vi "LJM logger write program config.vi"(0 "Working Directory":path, 7 "filename":string="ljstreamud.cfg", 9 "Program Configs":T1={"Data File Prefix"="", "Scan Rate (Hz)"=0.0, "Graph History"=0, "# Channels"=0, "Disable Scaling"=FALSE, "Max File Size (Bytes)"=0, "Channel Setup"={"Name"=["AIN0", "AIN1", "AIN2", "AIN3", "AIN4", "AIN5", "AIN6", "AIN7", "AIN8", "AIN9", "AIN10", "AIN11", "AIN12", "AIN13", "AIN14", "AIN15"], "", "Scaling Equation"=["y=a", "y=b", "y=c", "y=d", "y=e", "y=f", "y=g", "y=h", "y=i", "y=j", "y=k", "y=l", "y=m", "y=n", "y=o", "y=p"], "", "Graph?"=[TRUE, TRUE, TRUE, TRUE, FALSE, FALSE, FALSE, FALSE, FALSE, FALSE, FALSE, FALSE, FALSE, FALSE, FALSE, FALSE]}, "Interval (ms)"=0, "Write To File"=FALSE, "Log Every n Scans"=0}, 13 "Resolution":u8, 14 "SettlingFactor":u8) -> (15 "error out":errorcluster)   [LabVIEW 2026]
uses:
  Common Logger Controls/Program Config Cluster.ctl
  Common Logger Controls/Channel Setup.ctl
  <vilib>/Utility/config.llb/Write Key (String).vi
  <vilib>/Utility/config.llb/Write Key (I32).vi
  <vilib>/Utility/config.llb/Write Key (U32).vi
  <vilib>/Utility/config.llb/Write Key (Double).vi
  <vilib>/Utility/config.llb/Write Key (Boolean).vi
  <vilib>/Utility/config.llb/NI_LVConfig.lvlib
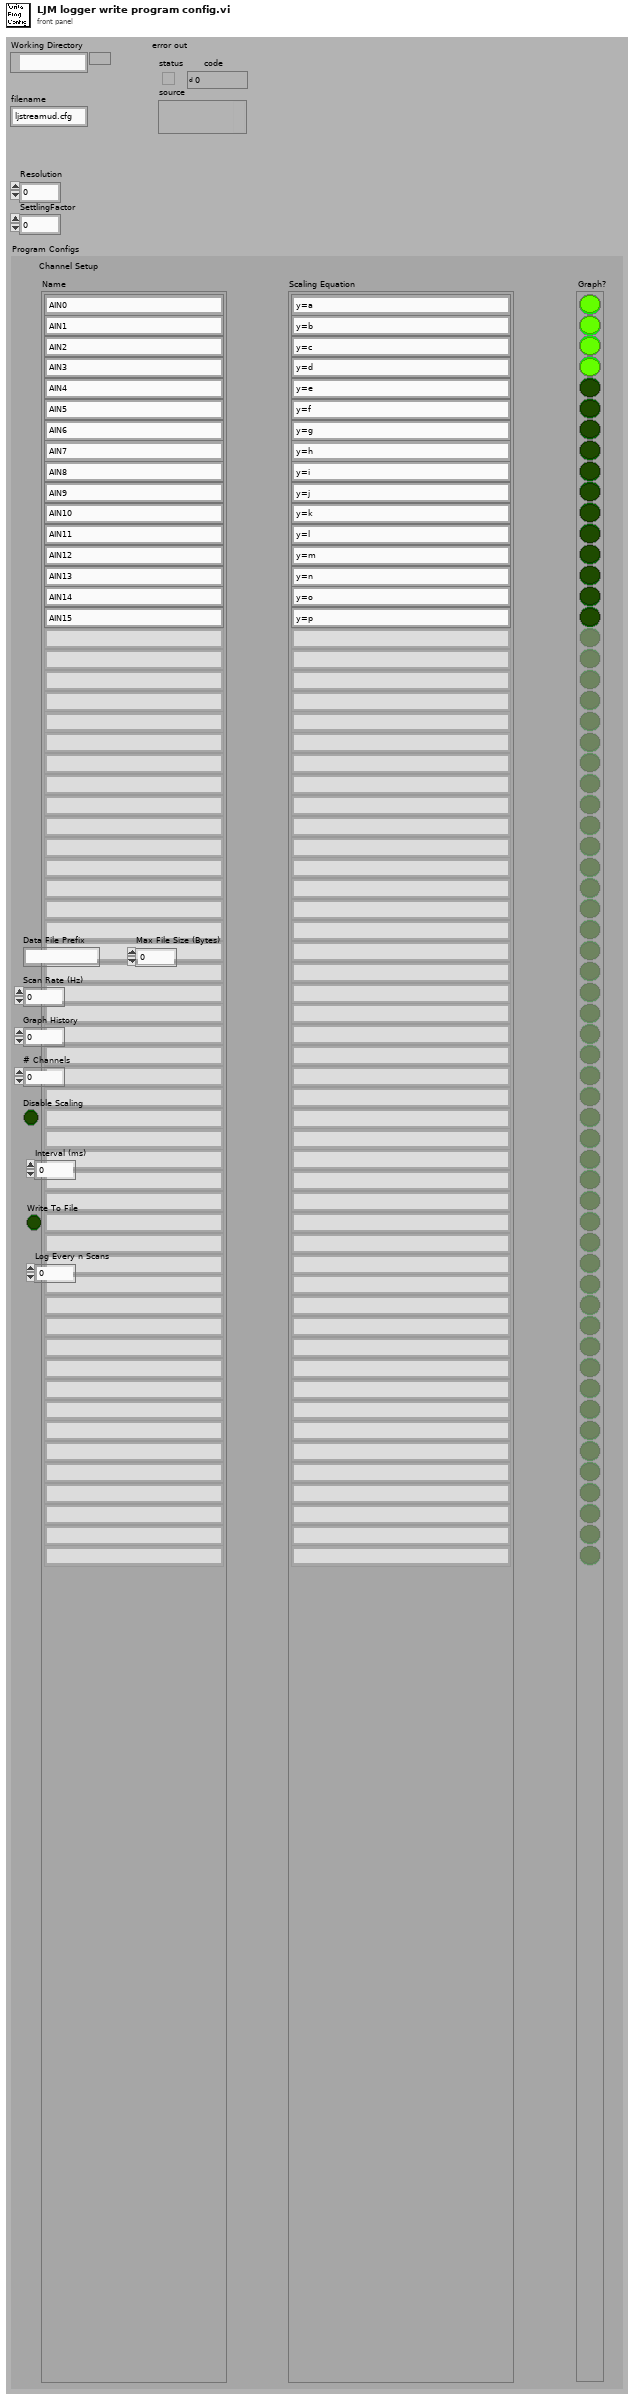
[diagram p1: front panel]
types:
  T1 = typedef "Program Config Cluster.ctl" = cluster{"Data File Prefix":string, "Scan Rate (Hz)":dbl, "Graph History":i32, "# Channels":i32, "Disable Scaling":bool, "Max File Size (Bytes)":i32, "Channel Setup":T2, "Interval (ms)":u32, "Write To File":bool, "Log Every n Scans":i32}
  T2 = typedef "Channel Setup.ctl" = cluster{"Name":string[], string, "Scaling Equation":string[], string, "Graph?":bool[]}
  T3 = typedef "NI_LVConfig.lvlib/Config Data RefNum.ctl" = refnum<k1>
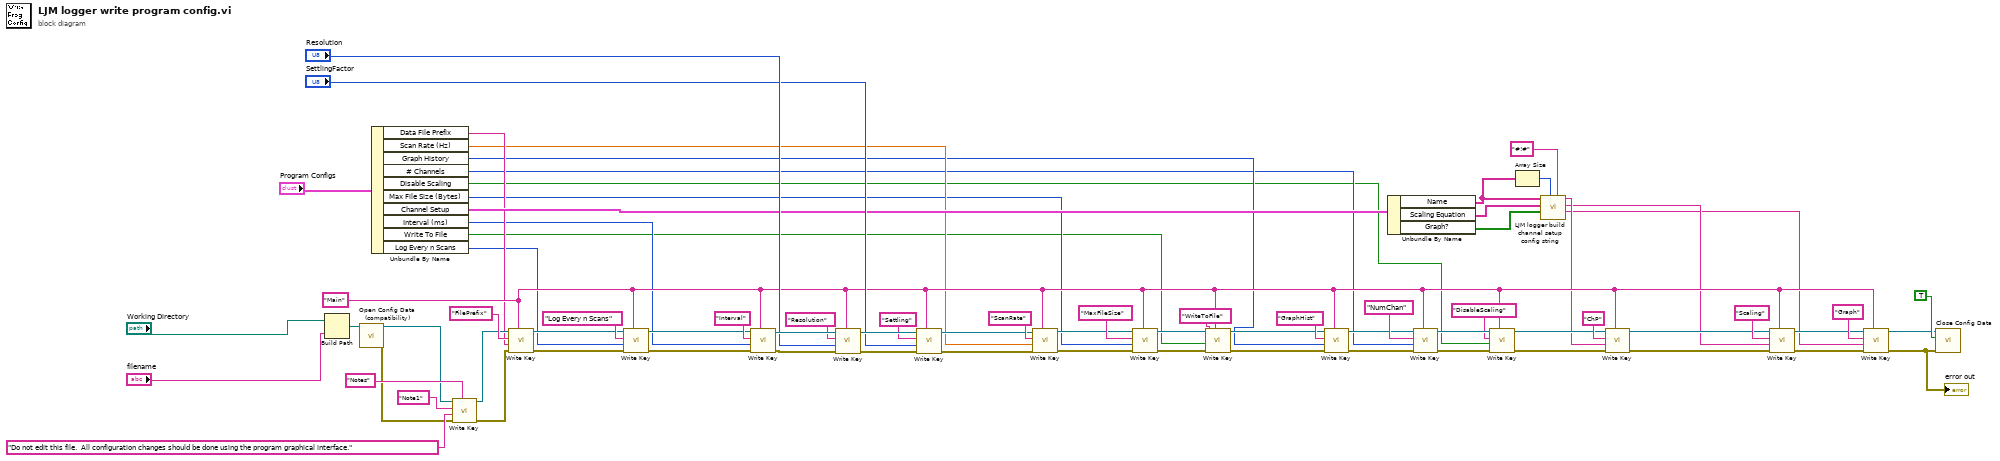
[diagram p0: block diagram]
diagram:
  w26 = "Main" ("section")
  n1 = Build Path(base path="Working Directory", name or relative path="filename") -> (appended path=w75:path)
  n2 = call <vilib>:"Open Config Data (compatibility).vi"("configuration file path"=w75) -> ("error out"=w28:errorcluster, "refnum"=w31:T3)  [unwired: 8 in, 1 out]
  n3 = Unbundle By Name("Program Configs") -> ("Data File Prefix"=w17:string, "Scan Rate (Hz)"=w14:dbl, "Graph History"=w11:i32, "# Channels"=w10:i32, "Disable Scaling"=w9:bool, "Max File Size (Bytes)"=w13:i32, "Channel Setup"=w18:T2, "Interval (ms)"=w15:u32, "Write To File"=w12:bool, "Log Every n Scans"=w16:i32)
  n4 = call-poly <vilib>:"Write Key.vi"("section"="Notes", "error in (no error)"=w28, "value"="Do not edit this file.  All configuration changes should be done using the program graphical interface." ("key"), "key"="Note1", "refnum"=w31) -> ("error out"=w29:errorcluster, "refnum out"=w30:T3)  [unwired: 4 in, 1 out]
  n5 = call-poly <vilib>:"Write Key.vi"("section"=w26, "error in (no error)"=w29, "value"=w17, "key"="FilePrefix", "refnum"=w30) -> ("error out"=w23:errorcluster, "refnum out"=w24:T3)  [unwired: 4 in, 1 out]
  n6 = call-poly <vilib>:"Write Key.vi"("section"=w26, "error in (no error)"=w23, "value"=w16, "key"="Log Every n Scans", "refnum"=w24) -> ("error out"=w22:errorcluster, "refnum out"=w25:T3)  [unwired: 4 in, 1 out]
  n7 = call-poly <vilib>:"Write Key.vi"("section"=w26, "error in (no error)"=w22, "value"=w15, "key"="Interval", "refnum"=w25) -> ("error out"=w53:errorcluster, "refnum out"=w52:T3)  [unwired: 4 in, 1 out]
  n8 = call-poly <vilib>:"Write Key.vi"("section"=w26, "error in (no error)"=w53, "value"="Resolution", "key"="Resolution", "refnum"=w52) -> ("error out"=w55:errorcluster, "refnum out"=w54:T3)  [unwired: 4 in, 1 out]
  n9 = call-poly <vilib>:"Write Key.vi"("section"=w26, "error in (no error)"=w55, "value"="SettlingFactor", "key"="Settling", "refnum"=w54) -> ("error out"=w45:errorcluster, "refnum out"=w46:T3)  [unwired: 4 in, 1 out]
  n10 = call-poly <vilib>:"Write Key.vi"("section"=w26, "error in (no error)"=w45, "value"=w14, "key"="ScanRate", "refnum"=w46) -> ("error out"=w42:errorcluster, "refnum out"=w41:T3)  [unwired: 4 in, 1 out]
  n11 = call-poly <vilib>:"Write Key.vi"("section"=w26, "error in (no error)"=w42, "value"=w13, "key"="MaxFileSize", "refnum"=w41) -> ("error out"=w38:errorcluster, "refnum out"=w39:T3)  [unwired: 4 in, 1 out]
  n12 = call-poly <vilib>:"Write Key.vi"("section"=w26, "error in (no error)"=w38, "value"=w12, "key"="WriteToFile", "refnum"=w39) -> ("error out"=w36:errorcluster, "refnum out"=w37:T3)  [unwired: 4 in, 1 out]
  n13 = call-poly <vilib>:"Write Key.vi"("section"=w26, "error in (no error)"=w36, "value"=w11, "key"="GraphHist", "refnum"=w37) -> ("error out"=w70:errorcluster, "refnum out"=w71:T3)  [unwired: 4 in, 1 out]
  n14 = Unbundle By Name(w18) -> ("Name"=w2:string[], "Scaling Equation"=w7:string[], "Graph?"=w6:bool[])
  n15 = call-poly <vilib>:"Write Key.vi"("section"=w26, "error in (no error)"=w70, "value"=w10, "key"="NumChan", "refnum"=w71) -> ("error out"=w65:errorcluster, "refnum out"=w66:T3)  [unwired: 4 in, 1 out]
  n16 = call-poly <vilib>:"Write Key.vi"("section"=w26, "error in (no error)"=w65, "value"=w9, "key"="DisableScaling", "refnum"=w66) -> ("error out"=w64:errorcluster, "refnum out"=w63:T3)  [unwired: 4 in, 1 out]
  n17 = Array Size(array=w2) -> (size(s)=w1:i32)
  n18 = call "LJM logger build channel setup config string.vi"("delimiter (#!#)"="#!#" ("delimiter (Tab)"), "Max Num Elements"=w1, "Bool list"=w6, "String list 2"=w7, "String list 1"=w2) -> ("Bool formatted"=w3:string, "String 2 formatted"=w4:string, "String 1 formatted"=w5:string)  [unwired: 3 in, 1 out]
  n19 = call-poly <vilib>:"Write Key.vi"("section"=w26, "error in (no error)"=w64, "value"=w5, "key"="ChP", "refnum"=w63) -> ("error out"=w20:errorcluster, "refnum out"=w21:T3)  [unwired: 4 in, 1 out]
  n20 = call-poly <vilib>:"Write Key.vi"("section"=w26, "error in (no error)"=w20, "value"=w4, "key"="Scaling", "refnum"=w21) -> ("error out"=w60:errorcluster, "refnum out"=w59:T3)  [unwired: 4 in, 1 out]
  n21 = call-poly <vilib>:"Write Key.vi"("section"=w26, "error in (no error)"=w60, "value"=w3, "key"="Graph", "refnum"=w59) -> ("error out"=w56:errorcluster, "refnum out"=w58:T3)  [unwired: 4 in, 1 out]
  "error out" <- w56
  n22 = call <vilib>:"Close Config Data.vi"("error in (no error)"=w56, "write file if changed (T)"=TRUE ("write configuration file? (F)"), "refnum"=w58) -> ()  [unwired: 7 in, 2 out]
